vi "test VISA.vi"() -> ()   [LabVIEW 2019]
uses:
  Controls/UDP - Command.ctl
  Controls/Communication - Write Data.ctl
panel:
  out "error out 2":errorcluster
  out "error out":errorcluster
  in  "Data":T1={"Test"={"Target Load"=0.0, "Target Disp"=0.0, "Rate"=0.0, "Speed"=0.0}, "Sensor"={"Name"=[], "Unit"=[], "Decimal Point"=[], "Ch Log"=[], "H Alarm"=[], "L Alarm"=[], "H Limit"=[], "L Limit"=[], "Filter"=[], "Gain"=[], "Calib Type"=[]}, "PID"={"SP"=0.0, "PV"=0.0, "kP"=0.0, "kI"=0.0, "kD"=0.0, "FF"=0.0, "Err Band"=0.0, "Max"=0, "Min"=0, "Ts"=0, "Out"=0, "Mode"=0}, "ADC"={"Active Ch"=[], "Filter Type"=0, "Post Filter"=[], "Gain"=[], "FS"=0, "IntOC"=0, "IntFC"=0, "SysOC"=0, "Cofficient"=[], "K"=[], "Max"=0}, "System"={"Out Type"=0, "Inverse"=0, "Monitor"=0, "Reserve"=0, "ACC Time"=0, "Pulse Rev"=0, "Stroke"=0, "Auto Off"=0, "Gear Ratio"=0.0, "Pitch"=0.0, "Max Speed"=0, "Jog Speed"=0, "Disp Coff"=0.0, "Max Load"=0}, "Index"=enum."Ch1", "Datalog"=enum."Empty"}
  out "Success":bool
  out "Data Channel":T2
  out "Data Unit":T3
  out "Raw Result":u8[](array[numeric])
  in  "Action":T4
  in  "VISA resource name":refnum<visa-resource-name>="COM6"
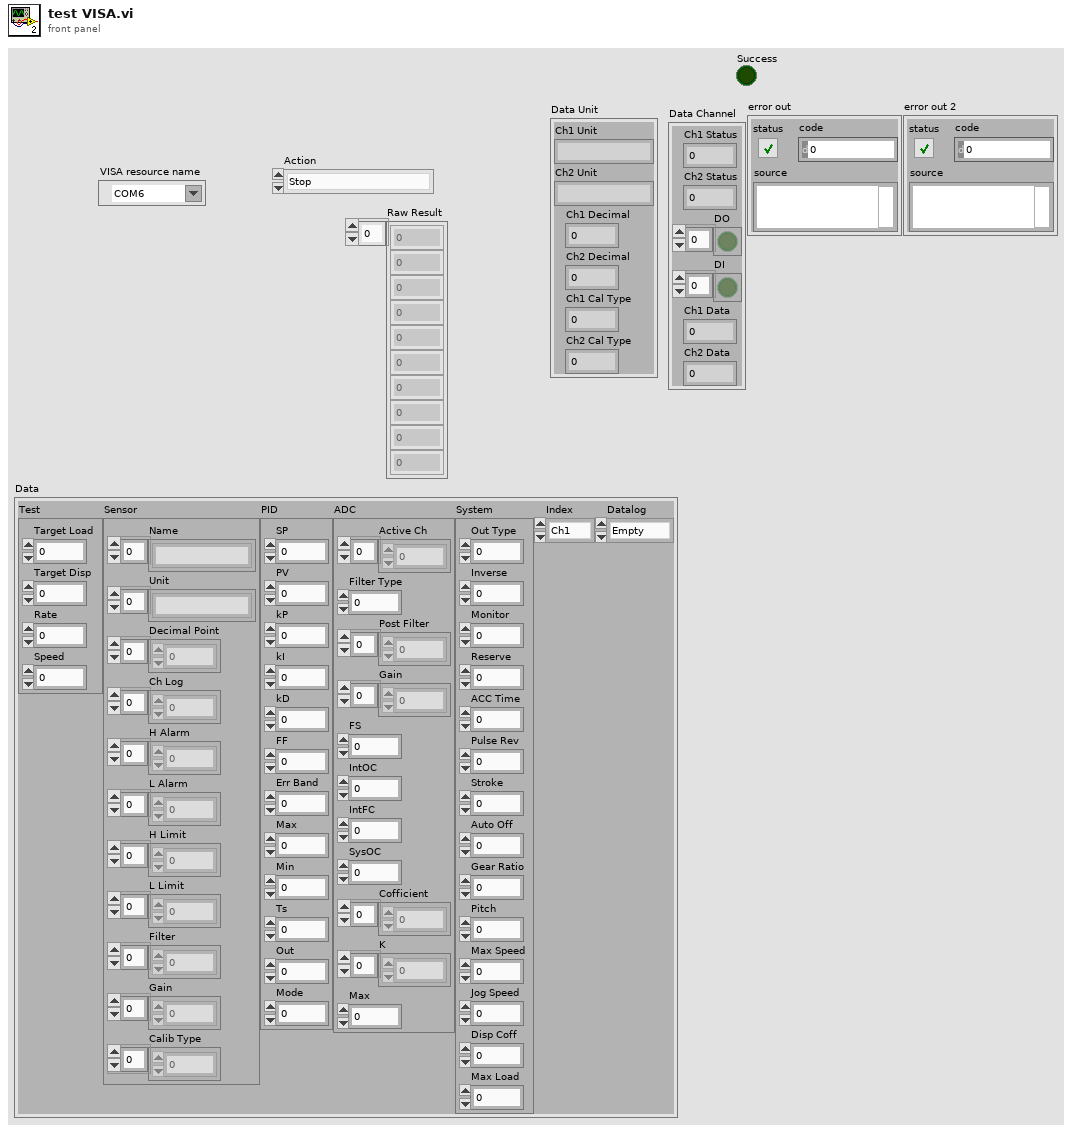
[diagram p1: front panel]
types:
  T1 = typedef "Communication - Write Data.ctl" = cluster{"Test":cluster{"Target Load":sgl, "Target Disp":sgl, "Rate":sgl, "Speed":sgl}, "Sensor":cluster{"Name":string[], "Unit":string[], "Decimal Point":u8[], "Ch Log":u8[], "H Alarm":u8[], "L Alarm":u8[], "H Limit":sgl[], "L Limit":sgl[], "Filter":u8[], "Gain":u8[], "Calib Type":u32[]}, "PID":cluster{"SP":sgl, "PV":sgl, "kP":sgl, "kI":sgl, "kD":sgl, "FF":sgl, "Err Band":sgl, "Max":i32, "Min":i32, "Ts":u32, "Out":i32, "Mode":u8}, "ADC":cluster{"Active Ch":u8[], "Filter Type":u8, "Post Filter":u8[], "Gain":u8[], "FS":u16, "IntOC":u8, "IntFC":u8, "SysOC":u8, "Cofficient":dbl[], "K":dbl[], "Max":i32}, "System":cluster{"Out Type":u8, "Inverse":u8, "Monitor":u8, "Reserve":u8, "ACC Time":u32, "Pulse Rev":u32, "Stroke":u32, "Auto Off":u32, "Gear Ratio":sgl, "Pitch":sgl, "Max Speed":u32, "Jog Speed":u32, "Disp Coff":sgl, "Max Load":u32}, "Index":enum16{"Ch1", "Ch2", "Ch3", "Ch4", "Ch5", "Ch6", "Ch7", "Ch8", "Ch9", "Ch10", "Ch11", "Ch12", "Ch13", "Ch14", "Ch15", "Ch16"}, "Datalog":enum16{"Ch1-Ch16", "Ch17-Ch32", "Ch32-Ch48", "Ch49-Ch64", "Empty"}}
  T2 = cluster{"Ch1 Status":u8, "Ch2 Status":u8, "DO":bool[], "DI":bool[], "Ch1 Data":sgl, "Ch2 Data":sgl}
  T3 = cluster{"Ch1 Unit":string, "Ch2 Unit":string, "Ch1 Decimal":u8, "Ch2 Decimal":u8, "Ch1 Cal Type":u8, "Ch2 Cal Type":u8}
  T4 = typedef "UDP - Command.ctl" = enum16{"Stop", "Jog Up", "Jog Down", "Ramp Up", "Ramp Down", "PID Target", "PID Ramp", "Disp Run", "Read Ch Data", "Zero Channel", "Zero Disp", "Read Sensor", "Write Sensor", "Read ADC", "Write ADC", "Read PID", "Write PID", "Read Test", "Write Test", "Read System", "Write System", "Read Datalog", "Read Datalog Sensor"}
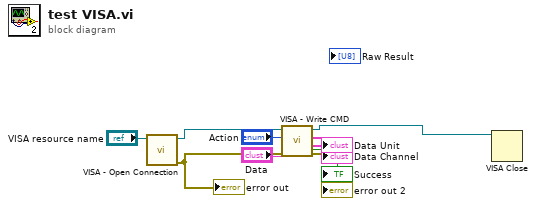
[diagram p0: block diagram]
diagram:
  n1 = call "VISA - Open Connection.vi"("VISA resource name"="VISA resource name") -> ("error out"=w10:errorcluster, "VISA Ref"=w9:refnum<visa-resource-name>)  [unwired: 9 in]
  "error out" <- w10
  n2 = call "VISA - Write CMD.vi"("error in"=w10, "Data"="Data", "Action"="Action", "VISA ref"=w9) -> ("error out"=→"error out 2":errorcluster, "Data Unit"=→"Data Unit":T3, "Data Channel"=→"Data Channel":T2, "VISA ref out"=w3:refnum<visa-resource-name>, "Success"=→"Success":bool)  [unwired: 1 in, 2 out]
  n3 = VISA Close(VISA resource name=w3) -> ()  [unwired: 1 in, 1 out]
